vi "Menu Init.vi"(8 "error in (no error)":errorcluster, 11 "IDE simple in":refnum<class "Main Panel.lvclass">) -> (0 "error out":errorcluster, 3 "IDE simple out":refnum<class "Main Panel.lvclass">)   [LabVIEW 2018, in "Main Panel.lvlib" / "Main Panel.lvclass"]
uses:
  Main Panel.lvclass
  Main Panel.lvclass/Main Panel.ctl
  <userlib>/_MGI/Menu Building/MenuTypes/Vi/VI.vi
  <userlib>/_MGI/Menu Building/MenuTypes/Vi/MGI_VI.lvclass
  <userlib>/_MGI/Menu Building/MenuTypes/MGI_Menu.lvclass
  Framework/Framework/Framework.lvclass
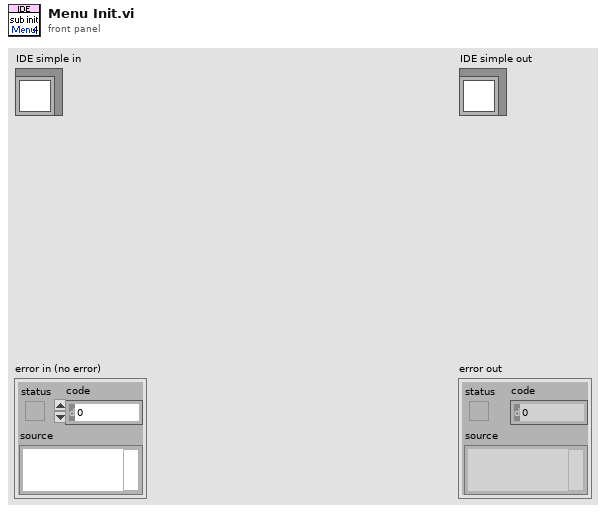
[diagram p1: front panel]
types:
  T1 = typedef "Framework.lvlib/Framework.lvclass/Const Lang Setting.ctl" = cluster{"Main Panel":T2, "Configuration Window":T15}
  T2 = typedef "Framework.lvlib/Framework.lvclass/Const Lang MainWnd.ctl" = cluster{"Title":T3, "Frame Basic":T5, "Frame Skill":T6, "bp":T7, "w":T8, "b":T9, "i":T10, "o":T11, "c":T12, "Other":T13, "Menu":T14}
  T3 = typedef "Framework.lvlib/Framework.lvclass/Const Lang MainWnd Frame Title.ctl" = cluster{"Frame Num":T4, "Name":T4}
  T4 = typedef "Framework.lvlib/Framework.lvclass/Const Lang Property.ctl" = cluster{"Name":string, "Tip":string, "Description":string}
  T5 = typedef "Framework.lvlib/Framework.lvclass/Const Lang MainWnd Frame Basic.ctl" = cluster{"pic":T4, "state":T4, "wait":T4, "next":T4, "dvx":T4, "dvy":T4, "dvz":T4, "centerx":T4, "centery":T4, "sound":T4}
  T6 = typedef "Framework.lvlib/Framework.lvclass/Const Lang MainWnd Frame Skill.ctl" = cluster{"mp":T4, "hit_a":T4, "hit_d":T4, "hit_j":T4, "hit_Fa":T4, "hit_Ua":T4, "hit_Da":T4, "hit_Fj":T4, "hit_Uj":T4, "hit_Dj":T4, "hit_ja":T4}
  T7 = typedef "Framework.lvlib/Framework.lvclass/Const Lang MainWnd Frame bp.ctl" = cluster{"x":T4, "y":T4}
  T8 = typedef "Framework.lvlib/Framework.lvclass/Const Lang MainWnd Frame w.ctl" = cluster{"kind":T4, "x":T4, "y":T4, "weaponact":T4, "cover":T4, "dvx":T4, "dvy":T4, "dvz":T4, "attacking":T4}
  T9 = typedef "Framework.lvlib/Framework.lvclass/Const Lang MainWnd Frame b.ctl" = cluster{"kind":T4, "x":T4, "y":T4, "w":T4, "h":T4, "index":T4}
  T10 = typedef "Framework.lvlib/Framework.lvclass/Const Lang MainWnd Frame i.ctl" = cluster{"kind":T4, "x":T4, "y":T4, "w":T4, "h":T4, "zwidth":T4, "dvx":T4, "dvy":T4, "dvz":T4, "fall":T4, "arest":T4, "vrest":T4, "bdefend":T4, "injury":T4, "effect":T4, "catchingact 1":T4, "catchingact 2":T4, "caughtact 1":T4, "caughtact 2":T4, "index":T4}
  T11 = typedef "Framework.lvlib/Framework.lvclass/Const Lang MainWnd Frame o.ctl" = cluster{"kind":T4, "x":T4, "y":T4, "action":T4, "dvx":T4, "dvy":T4, "dvz":T4, "oid":T4, "facing":T4}
  T12 = typedef "Framework.lvlib/Framework.lvclass/Const Lang MainWnd Frame c.ctl" = cluster{"kind":T4, "x":T4, "y":T4, "injury":T4, "cover":T4, "vaction":T4, "aaction":T4, "taction":T4, "hurtable":T4, "decrease":T4, "fronthurtact":T4, "backhurtact":T4, "throwvx":T4, "throwvy":T4, "throwvz":T4, "throwinjury":T4, "dircontrol":T4}
  T13 = typedef "Framework.lvlib/Framework.lvclass/Const Lang MainWnd Other.ctl" = cluster{"File Path":T4, "GoTo":T4, "Apply Change":T4, "To Next Frame":T4, "Sound Play":T4}
  T14 = typedef "Framework.lvlib/Framework.lvclass/Const Lang MainWnd Menu.ctl" = cluster{"File":T4, "Open File":T4, "Save File":T4, "Exit":T4, "Settings":T4, "Preferences":T4, "Help":T4, "Show Context Help":T4}
  T15 = typedef "Framework.lvlib/Framework.lvclass/Const Lang CfgWnd.ctl" = cluster{"Tab":T16, "Main":T17, "Path":T18, "Image":T19}
  T16 = typedef "Framework.lvlib/Framework.lvclass/Const Lang CfgWnd Tab.ctl" = cluster{"Main Page":T4, "Image Page":T4}
  T17 = typedef "Framework.lvlib/Framework.lvclass/Const Lang CfgWnd Main.ctl" = cluster{"Language":T4, "Save":T4, "Cancel":T4}
  T18 = typedef "Framework.lvlib/Framework.lvclass/Const Lang CfgWnd Path.ctl" = cluster{"Reset":T4, "Path Data":T4, "Path Png":T4, "Path Mp3":T4}
  T19 = typedef "Framework.lvlib/Framework.lvclass/Const Lang CfgWnd Image.ctl" = cluster{"Center Point":cluster{"Name":T4, "Size":T4, "Color":T4, "Enable":T4}, "bp Point":cluster{"Name":T4, "Size":T4, "Color":T4, "Enable":T4}, "w Point":cluster{"Name":T4, "Size":T4, "Color":T4, "Enable":T4}, "b Box":cluster{"Name":T4, "Fill Color":T4, "Border Color":T4, "Enable":T4}, "i Box":cluster{"Name":T4, "Fill Color":T4, "Border Color":T4, "Enable":T4}, "o Point":cluster{"Name":T4, "Size":T4, "Color":T4, "Enable":T4}, "c Point":cluster{"Name":T4, "Size":T4, "Color":T4, "Enable":T4}}
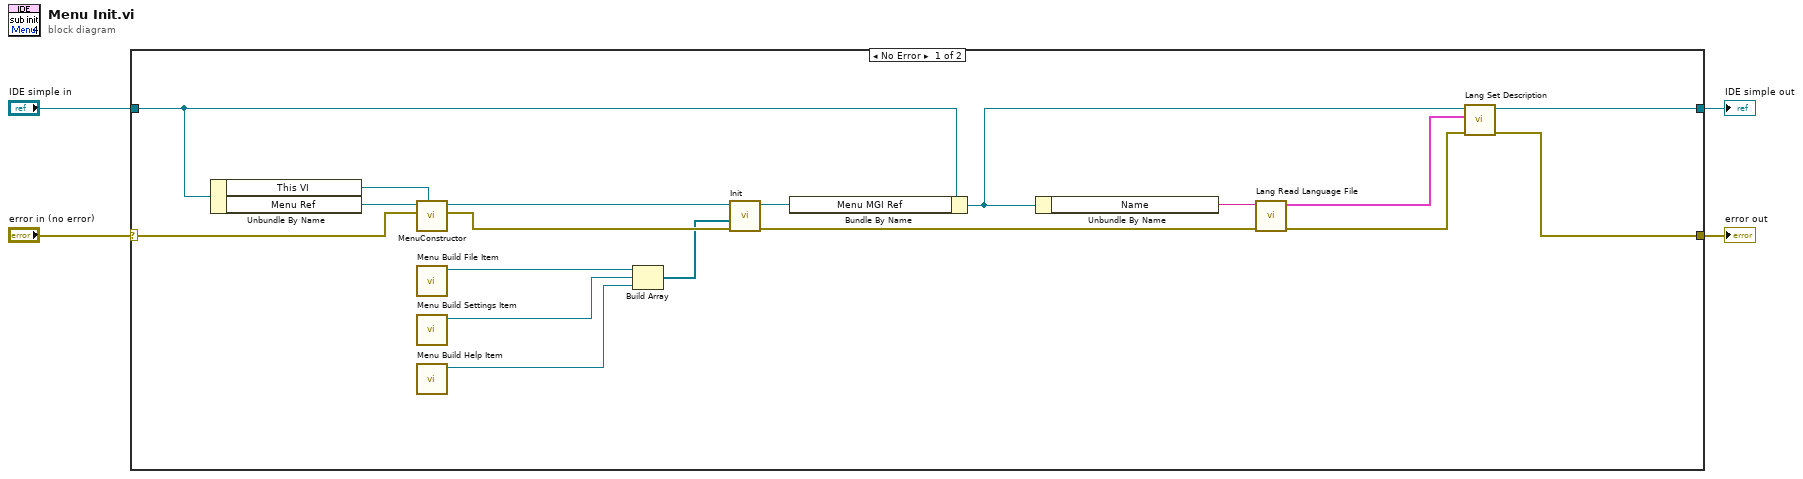
[diagram p0: block diagram]
diagram:
  n1 = case shown="No Error" "error in (no error)" {
    selector: "error in (no error)" -> [w19 w24]
    tunnel: [w5 w24] -> w3
    tunnel: [w6 w23] -> w1
    tunnel: "IDE simple in" -> [w20 w23]
    frame No Error {
      n2 = Unbundle By Name(w20) -> ("This VI"=w21:refnum<vi>, "Menu Ref"=w22:refnum<k9>)
      n3 = call-poly <userlib>:"MenuConstructor.vi"("Menu VI"=w21, "error in (no error)"=w19, "menu reference"=w22) -> ("error out"=w18:errorcluster, "VI"=w17:refnum<class "MGI_VI.lvclass">)  [unwired: 7 in]
      n4 = call "Menu Build File Item.vi"() -> ("Menu File Item"=w16:refnum<data-value>)  [unwired: 11 in]
      n5 = call "Menu Build Settings Item.vi"() -> ("Menu Settings Item"=w14:refnum<data-value>)  [unwired: 11 in]
      n6 = call "Menu Build Help Item.vi"() -> ("Menu Settings Item"=w12:refnum<data-value>)  [unwired: 11 in]
      n7 = Build Array(w16, w14, w12) -> (w15:refnum<data-value>[])
      n8 = call-dynamic "Init.vi"("error in (no error)"=w18, "Menu Items"=w15, "Menu in"=w17) -> ("error out"=w8:errorcluster, "Menu out"=w13:refnum<class "MGI_VI.lvclass">)  [unwired: 6 in, 1 out]
      n9 = Bundle By Name(cluster=w20, "Menu MGI Ref"=w13) -> (w7:refnum<class "Main Panel.lvclass">)
      n10 = Unbundle By Name(w7) -> ("Name"=w10:string)
      n11 = call "Lang Read Language File.vi"("error in (no error)"=w8, "Language Name"=w10) -> ("error out"=w11:errorcluster, "UI Descriptions"=w9:T1)  [unwired: 7 in, 1 out]
      n12 = call "Lang Set Description.vi"("error in (no error)"=w11, "UI Descriptions"=w9, "LF2R IDE in"=w7) -> ("error out"=w5:errorcluster, "LF2R IDE out"=w6:refnum<class "Main Panel.lvclass">)  [unwired: 7 in]
    }
    frame Error {
    }
  }
  "error out" <- w3
  "IDE simple out" <- w1
